vi "Convert Recipe Valve to Valve List.vi"(5 "Valves on Shared Lines":i32, 7 "Valves Per Reactor":i32, 9 "Number of Reactors":i32, 10 "Reactor ID#":i32, 13 "Valve Number":i32) -> (2 "Valve List":i32[](array[numeric]))   [LabVIEW 2022 SP3]
panel:
  out "Valves on Shared 1":i32
  out "Valves Per Reactor":i32
  out "Number of Reactors":i32
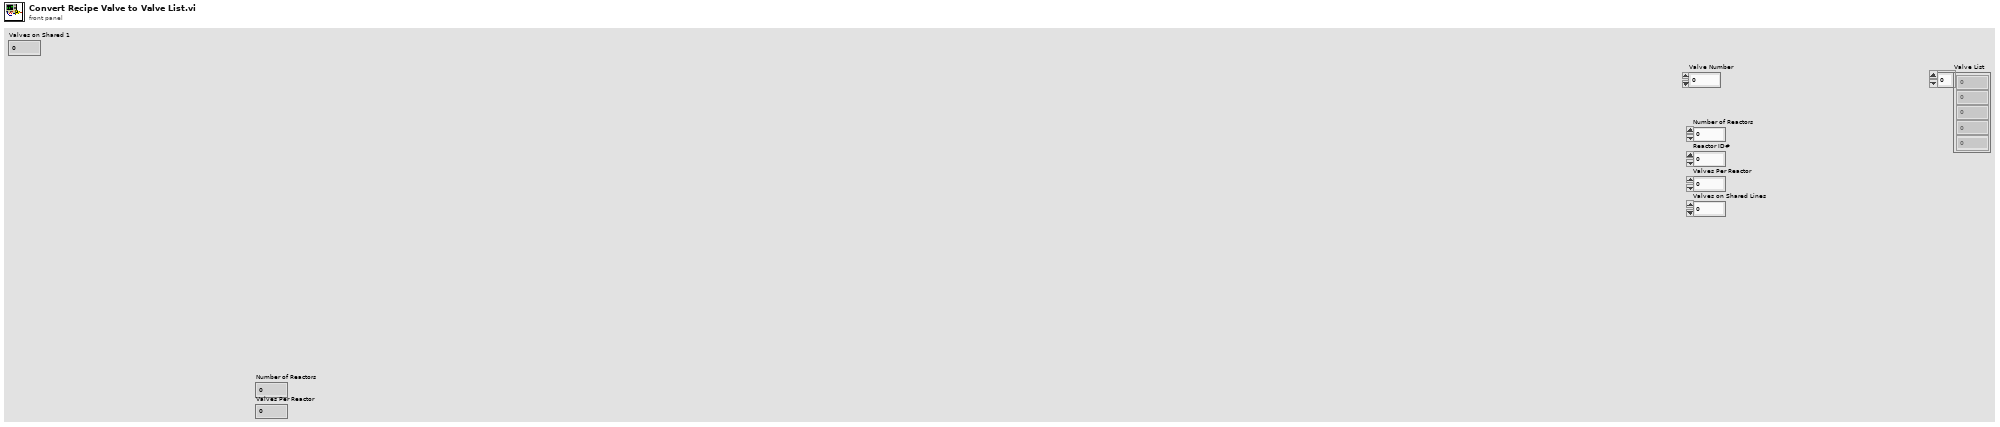
[diagram p1: front panel]
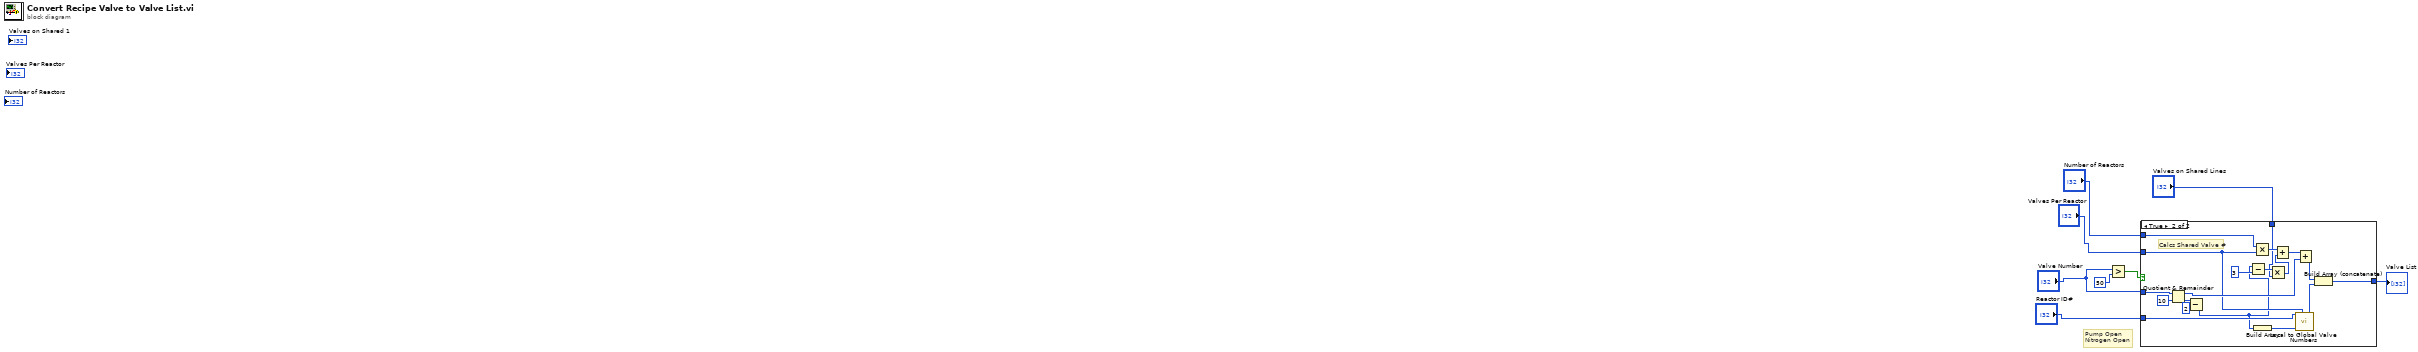
[diagram p0: block diagram]
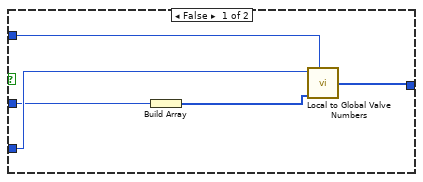
[diagram p2: hidden frame]
diagram:
  # "Pump Open\nNitrogen Open"
  n1 = Greater?(x="Valve Number", y=50 ("lower limit")) -> (0:w1:bool)
  n2 = case shown="True" w1 {
    tunnel: "Valve Number" -> [w10 w31]
    tunnel: "Number of Reactors" -> [_ w22]
    tunnel: "Valves Per Reactor" -> [w11 w20]
    tunnel: "Valves on Shared Lines" -> [_ w21]
    tunnel: "Reactor ID#" -> [w12 w19]
    tunnel: [w13 w14] -> w4
    frame False {
      n3 = Build Array(w10) -> (w9:i32[])
      n4 = call "Local to Global Valve Numbers.vi"("Reactor ID #"=w12, "List of Local Valves"=w9, "Valves Per Reactor"=w11) -> ("List of Global Valves"=w13:i32[])  [unwired: 2 in]
    }
    frame True {
      # "Calcs Shared Valve #"
      n5 = Quotient & Remainder(x=w31, y=10) -> (x-y*floor(x/y)=w23:i32, floor(x/y)=w30:i32)
      n6 = Subtract(x=w30, y=2) -> (x-y=w18:i32)
      n7 = Subtract(x=w18, y=3) -> (x-y=w26:i32)
      n8 = Multiply(x=w22, y=w20) -> (x*y=w25:i32)
      n9 = Build Array(w18) -> (w17:i32[])
      n10 = Multiply(x=w26, y=w21) -> (x*y=w27:i32)
      n11 = Add(x=w25, y=w27) -> (x+y=w28:i32)
      n12 = call "Local to Global Valve Numbers.vi"("Reactor ID #"=w19, "List of Local Valves"=w17, "Valves Per Reactor"=w20) -> ("List of Global Valves"=w15:i32[])  [unwired: 2 in]
      n13 = Add(x=w28, y=w23) -> (x+y=w16:i32)
      n14 = Build Array (concatenate)(w16, w15) -> (w14:i32[])
    }
  }
  "Valve List" <- w4
